vi "#22_MAV_MSG_PARAM_VALUE_DECODE.vi"(11 "mavlink_payload":u8[](array[numeric])) -> (3 "PARAM_VALUE":T1)   [LabVIEW 2023]
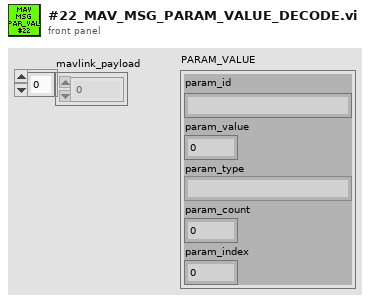
[diagram p1: front panel]
types:
  T1 = cluster{"param_id":string, "param_value":sgl, "param_type":enum16{"", "MAV_PARAM_TYPE_UINT8", "MAV_PARAM_TYPE_INT8", "MAV_PARAM_TYPE_UINT16", "MAV_PARAM_TYPE_INT16", "MAV_PARAM_TYPE_UINT32", "MAV_PARAM_TYPE_INT32", "MAV_PARAM_TYPE_UINT64", "MAV_PARAM_TYPE_INT64", "MAV_PARAM_TYPE_REAL32", "MAV_PARAM_TYPE_REAL64"}, "param_count":u16, "param_index":u16}
  T2 = enum16{"", "MAV_PARAM_TYPE_UINT8", "MAV_PARAM_TYPE_INT8", "MAV_PARAM_TYPE_UINT16", "MAV_PARAM_TYPE_INT16", "MAV_PARAM_TYPE_UINT32", "MAV_PARAM_TYPE_INT32", "MAV_PARAM_TYPE_UINT64", "MAV_PARAM_TYPE_INT64", "MAV_PARAM_TYPE_REAL32", "MAV_PARAM_TYPE_REAL64"}
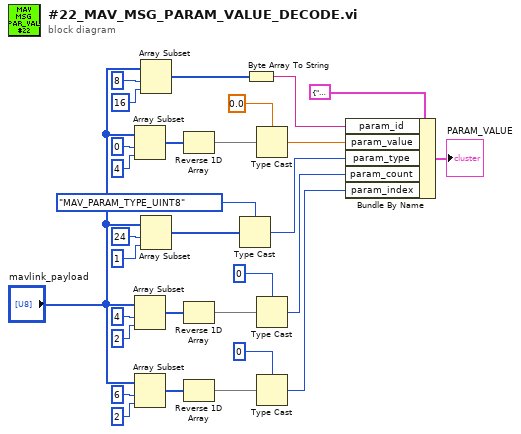
[diagram p0: block diagram]
diagram:
  n1 = Array Subset(array="mavlink_payload", index=0 ("Index"), length=4) -> (w26:u8[])
  n2 = Array Subset(array="mavlink_payload", index=4 ("Index"), length=2) -> (w15:u8[])
  n3 = Array Subset(array="mavlink_payload", index=6 ("Index"), length=2) -> (w9:u8[])
  n4 = Array Subset(array="mavlink_payload", index=8 ("Index"), length=16) -> (w2:u8[])
  n5 = Array Subset(array="mavlink_payload", index=24 ("Index"), length=1) -> (w20:u8[])
  n6 = Reverse 1D Array(array=w26) -> (reversed array=w25:u8[])
  n7 = Reverse 1D Array(array=w15) -> (reversed array=w14:u8[])
  n8 = Reverse 1D Array(array=w9) -> (reversed array=w8:u8[])
  n9 = Type Cast(type=T2."MAV_PARAM_TYPE_UINT8" ("param_type"), x=w20) -> (*(type *) &x=w19:T2)
  n10 = Byte Array To String(unsigned byte array=w2) -> (string=w1:string)
  n11 = Type Cast(type=sgl 0.0 ("Index"), x=w25) -> (*(type *) &x=w23:sgl)
  n12 = Type Cast(type=u16 0 ("Index"), x=w14) -> (*(type *) &x=w12:u16)
  n13 = Type Cast(type=u16 0 ("Index"), x=w8) -> (*(type *) &x=w6:u16)
  n14 = Bundle By Name(cluster=T1 {"param_id"="", "param_value"=0.0, "param_type"=enum."MAV_PARAM_TYPE_UINT8", "param_count"=0, "param_index"=0} ("PARAM_VALUE"), "param_id"=w1, "param_value"=w23, "param_type"=w19, "param_count"=w12, "param_index"=w6) -> (→"PARAM_VALUE":T1)
